vi "1.vi"() -> ()   [LabVIEW 2015]
panel:
  in  "OK Button":bool=TRUE
  in  "Requested Plots":T1(array[cluster])
  out "Waveform chart":waveform(dbl)[](graph)=[{"t0"=timestamp(3537897551.4112577 s since 1904-01-01), "dt"=1.0, "Y"=[1.0]}, {"t0"=timestamp(3537897551.411394 s since 1904-01-01), "dt"=1.0, "Y"=[52636.62109375]}, {"t0"=timestamp(3537897551.411678 s since 1904-01-01), "dt"=1.0, "Y"=[-339720.71875]}, {"t0"=timestamp(3537897551.411799 s since 1904-01-01), "dt"=1.0, "Y"=[202592.15625]}, {"t0"=timestamp(3537897551.4119 s since 1904-01-01), "dt"=1.0, "Y"=[-23028.4296875]}, {"t0"=timestamp(3537897551.411996 s since 1904-01-01), "dt"=1.0, "Y"=[88723.75]}, {"t0"=timestamp(3537897551.41212 s since 1904-01-01), "dt"=1.0, "Y"=[80100.75]}, {"t0"=timestamp(3537897551.310503 s since 1904-01-01), "dt"=1.0, "Y"=[-548105.4375]}]
  out "net address":u32
  out "port or service name":u16=5803
  in  "stop":bool
  out "error out":errorcluster
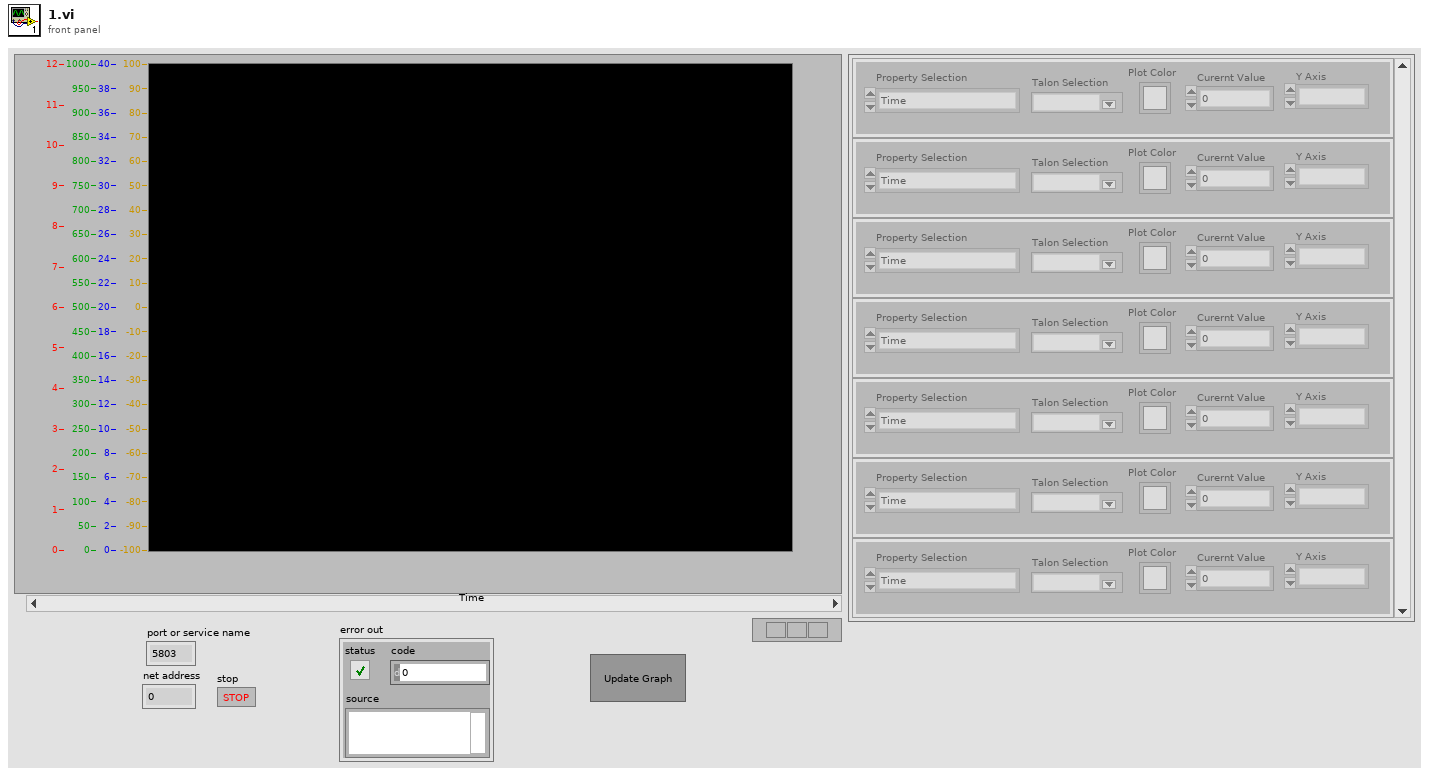
[diagram p1: front panel]
types:
  T1 = cluster{"Property Selection":enum16{"Time", "TalonID", "OutputVoltage", "OutputCurrent", "PIDError", "Encoder Position", "Encoder Velocity", "Commanded Value", "I Zone", "I Accumulation"}, "Talon Selection":u16, "Plot Color":u32, "Curernt Value":dbl, "New Current Value?":bool, "output waveform":waveform(dbl), "Y Axis":enum16{"Red Axis", "Green Axis", "Blue Axis", "Yellow Axis"}}[]
  T2 = enum16{"Red Axis", "Green Axis", "Blue Axis", "Yellow Axis"}[]
  T3 = enum16{"Time", "TalonID", "OutputVoltage", "OutputCurrent", "PIDError", "Encoder Position", "Encoder Velocity", "Commanded Value", "I Zone", "I Accumulation"}
  T4 = enum16{"Red Axis", "Green Axis", "Blue Axis", "Yellow Axis"}
  T5 = cluster{"Property Selection":enum16{"Time", "TalonID", "OutputVoltage", "OutputCurrent", "PIDError", "Encoder Position", "Encoder Velocity", "Commanded Value", "I Zone", "I Accumulation"}, "Talon Selection":u16, "Plot Color":u32, "Curernt Value":dbl, "New Current Value?":bool, "output waveform":waveform(dbl), "Y Axis":enum16{"Red Axis", "Green Axis", "Blue Axis", "Yellow Axis"}}
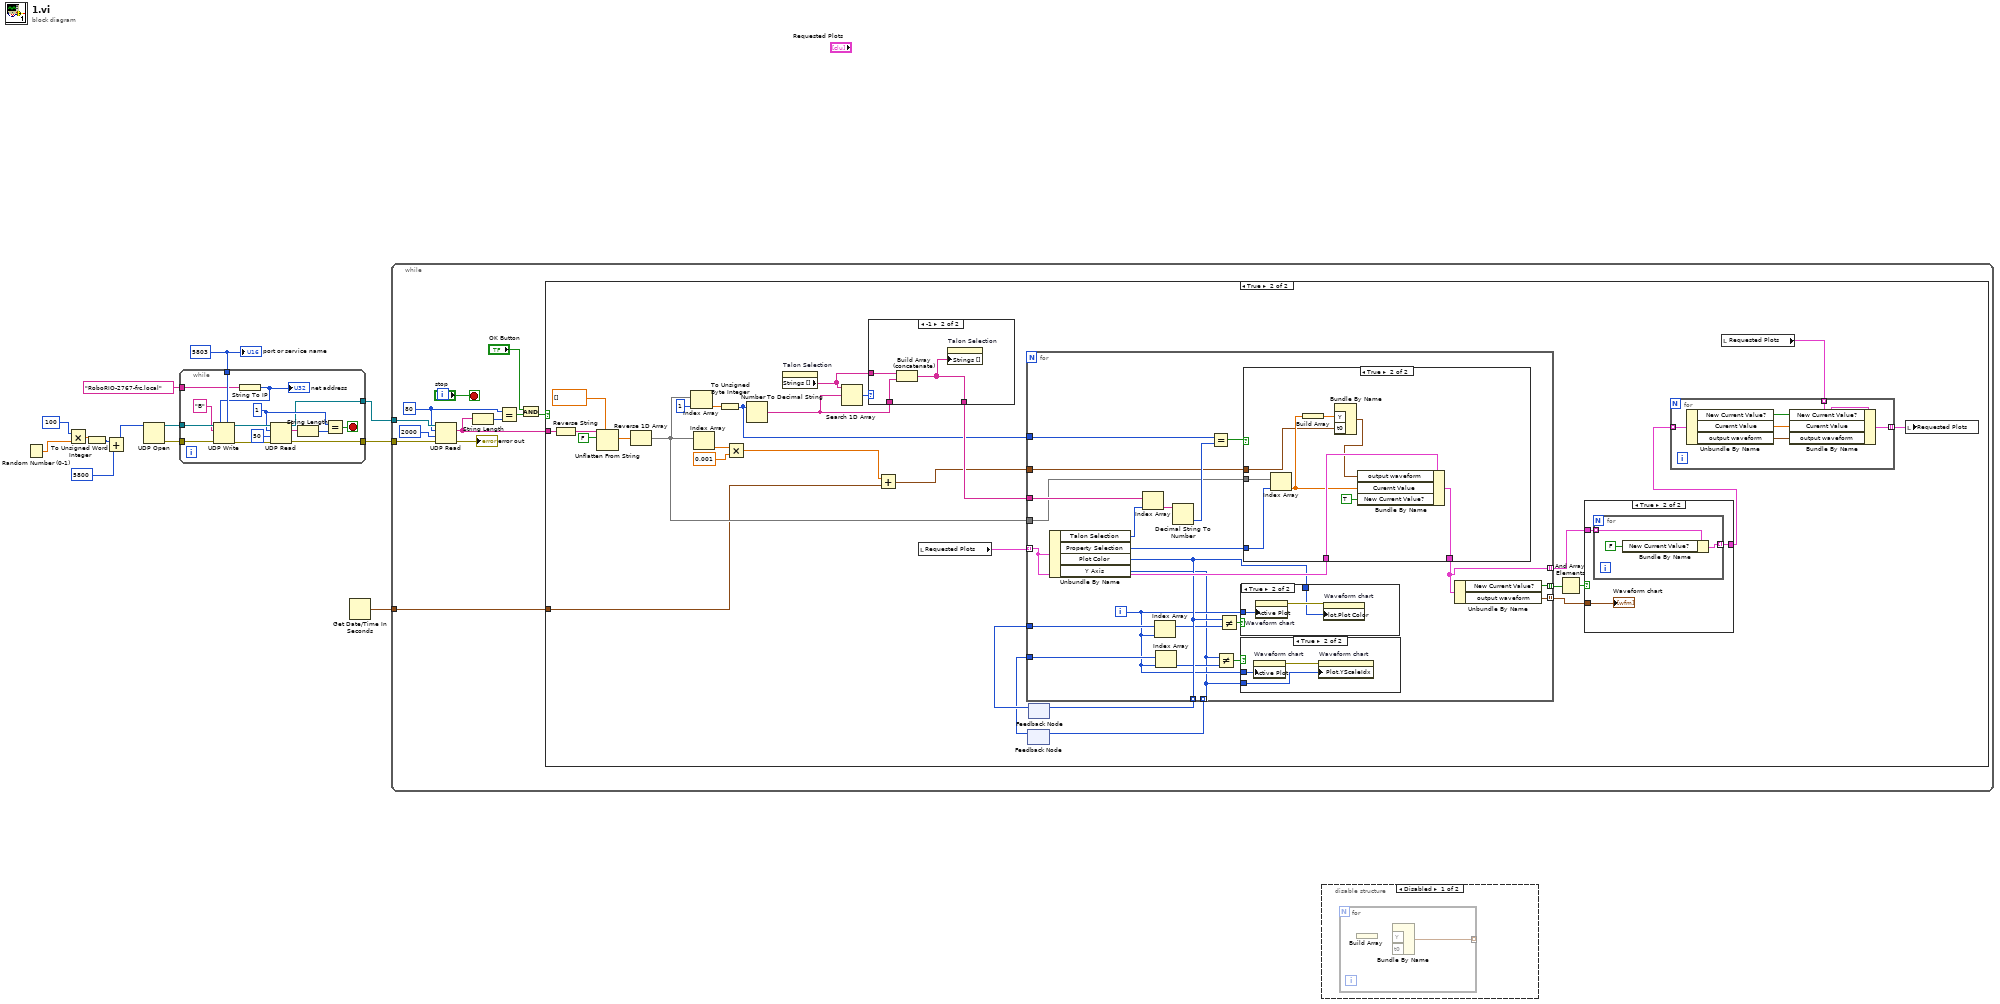
[diagram p0: block diagram]
diagram:
  w3 = u16 5803 ("port or service name")
  n1 = Random Number (0-1)() -> (number: 0 to 1=w7:dbl)
  n2 = Multiply(x=u16 100 ("port"), y=w7) -> (x*y=w6:dbl)
  n3 = To Unsigned Word Integer(number=w6) -> (unsigned 16bit integer=w5:u16)
  n4 = Add(x=w5, y=u16 5800 ("port")) -> (x+y=w9:u16)
  n5 = UDP Open(11:w9) -> (port=w13:refnum<k16>, 0:w12:errorcluster)  [unwired: 4 in, 1 out]
  n6 = while {
    tunnel: w13 -> [w28]
    tunnel: [w21] -> w4
    tunnel: w12 -> [w20]
    tunnel: [w19] -> w11
    tunnel: w3 -> [w17]
    tunnel: "RoboRIO-2767-frc.local" ("name") -> [w16]
    stop <- w22 stop-if-true
    w23 = 1 ("max size (548)")
    n7 = String To IP(1:w16) -> (0:w15:u32)
    "net address" <- w15
    n8 = UDP Write(address=w15, port or service name=w17, connection ID=w28, data in="B", 8:w20) -> (error out=w27:errorcluster, 3:w26:refnum<k16>)  [unwired: 1 in]
    n9 = UDP Read(connection ID=w26, max size (548)=w23, timeout ms (25000)=50, 8:w27) -> (data out=w25:string, error out=w19:errorcluster, 3:w21:refnum<k16>)  [unwired: 2 out]
    n10 = String Length(string=w25) -> (length=w24:i32)
    n11 = Equal?(x=w23, y=w24) -> (x = y?=w22:bool)
  }
  n12 = Get Date/Time In Seconds() -> (seconds since 1Jan1904=w1:timestamp)
  n13 = while {
    tunnel: w4 -> [w40]
    tunnel: w11 -> [w39]
    tunnel: w1 -> [w31]
    stop <- "stop" stop-if-true
    w33 = 80 ("max size (548)")
    n14 = UDP Read(connection ID=w40, max size (548)=w33, timeout ms (25000)=2000, 8:w39) -> (data out=w35:string, error out=→"error out":errorcluster)  [unwired: 3 out]
    n15 = String Length(string=w35) -> (length=w34:i32)
    n16 = Equal?(x=w33, y=w34) -> (x = y?=w32:bool)
    n17 = And(x="OK Button", y=w32) -> (x .and. y?=w30:bool)
    n18 = case shown="True" w30 {
      tunnel: w35 -> [_ w69]
      tunnel: w31 -> [_ w53]
      frame False {
      }
      frame True {
        n19 = Reverse String(1:w69) -> (0:w68:string)
        n20 = Unflatten From String(type=dbl[] [], binary string=w68, data includes array or string size? (T)=FALSE) -> (value=w66:dbl[])  [unwired: 2 in, 2 out]
        n21 = Reverse 1D Array(array=w66) -> (reversed array=w56:dbl[])
        n22 = Index Array(array=w56, index=1) -> (element=w62:dbl)
        n23 = Index Array(array=w56) -> (element=w65:dbl)  [unwired: 1 in]
        n24 = To Unsigned Byte Integer(number=w62) -> (unsigned 8bit integer=w57:u8)
        n25 = Multiply(x=w65, y=0.001) -> (x*y=w52:dbl)
        n26 = Number To Decimal String(number=w57) -> (decimal integer string=w59:string)  [unwired: 1 in]
        n27 = property on="Talon Selection" class="Ring (strict)"() -> ("Strings []"=w60:string[])  [unwired: 2 in, 2 out]
        n28 = Search 1D Array(1D array=w60, element=w59) -> (index of element=w61:i32)  [unwired: 1 in]
        n29 = case shown="-1" w61 {
          tunnel: w60 -> [w84 w86]
          tunnel: w59 -> [_ w87]
          tunnel: [w84 w85] -> w58
          frame 0, Default {
          }
          frame -1 {
            n30 = Build Array (concatenate)(w86, w87) -> (w85:string[])
            n31 = property on="Talon Selection" class="Ring (strict)"("Strings []"=w85) -> ()  [unwired: 2 in, 2 out]
          }
        }
        n32 = Add(x=w52, y=w53) -> (x+y=w54:timestamp)
        n33 = local read "Requested Plots"() -> (w49:T1)
        n34 = feedback #1() -> (w42:T2)  [unwired: 1 in]
        n35 = feedback #2() -> (w46:u32[])  [unwired: 1 in]
        n36 = for {
          tunnel: w49 -> [w101] mode=indexing
          tunnel: w58 -> [w108]
          tunnel: w57 -> [w106]
          tunnel: w56 -> [w102]
          tunnel: [w100] -> w55 mode=indexing
          tunnel: w54 -> [w99]
          tunnel: [w98] -> w50 mode=indexing
          tunnel: [w97] -> w48 mode=indexing
          tunnel: [w95] -> w47 mode=indexing
          tunnel: w46 -> [w93]
          tunnel: w42 -> [w92]
          tunnel: [w88] -> w41 mode=indexing
          i -> [w89]
          n37 = Unbundle By Name(w101) -> ("Talon Selection"=w109:u16, "Property Selection"=w103:T3, "Plot Color"=w95:u32, "Y Axis"=w88:T4)
          n38 = Index Array(array=w108, index=w109) -> (element=w107:string)
          n39 = Index Array(array=w93, index=w89) -> (element=w94:u32)
          n40 = Index Array(array=w92, index=w89) -> (element=w90:T4)
          n41 = Decimal String To Number(string=w107) -> (number=w105:i32)  [unwired: 2 in, 1 out]
          n42 = Equal?(x=w106, y=w105) -> (x = y?=w104:bool)
          n43 = Not Equal?(x=w88, y=w90) -> (x != y?=w91:bool)
          n44 = Not Equal?(x=w95, y=w94) -> (x != y?=w96:bool)
          n45 = case shown="True" w96 {
            tunnel: w89 -> [_ w114]
            tunnel: w95 -> [_ w113]
            frame False {
            }
            frame True {
              n46 = property on="Waveform chart" class="WFChart (strict)"("Active Plot"=w114) -> (error out=w115:errorcluster)  [unwired: 2 in, 1 out]
              n47 = property on="Waveform chart" class="WFChart (strict)"(error in=w115, "Plot.Plot Color"=w113) -> ()  [unwired: 1 in, 2 out]
            }
          }
          n48 = case shown="True" w91 {
            tunnel: w89 -> [_ w112]
            tunnel: w88 -> [_ w110]
            frame False {
            }
            frame True {
              n49 = property on="Waveform chart" class="WFChart (strict)"("Active Plot"=w112) -> (error out=w111:errorcluster)  [unwired: 2 in, 1 out]
              n50 = property on="Waveform chart" class="WFChart (strict)"(error in=w111, "Plot.YScaleIdx"=w110) -> ()  [unwired: 1 in, 2 out]
            }
          }
          n51 = case shown="True" w104 {
            tunnel: w103 -> [_ w124]
            tunnel: w102 -> [_ w125]
            tunnel: w101 -> [w116 w123]
            tunnel: [w116 w122] -> w97
            tunnel: w99 -> [_ w117]
            frame False {
            }
            frame True {
              n52 = Index Array(array=w125, index=w124) -> (element=w119:dbl)
              n53 = Build Array(w119) -> (w118:dbl[])
              n54 = Bundle By Name("Y"=w118, "t0"=w117) -> (w120:waveform(dbl))  [unwired: 1 in]
              n55 = Bundle By Name(cluster=w123, "output waveform"=w120, "Curernt Value"=w119, "New Current Value?"=TRUE) -> (w122:T5)
            }
          }
          n56 = Unbundle By Name(w97) -> ("New Current Value?"=w100:bool, "output waveform"=w98:waveform(dbl))
        }
        n57 = feedback-in #1(w41) -> ()
        n58 = feedback-in #2(w47) -> ()
        n59 = And Array Elements(Boolean array=w55) -> (logical AND=w51:bool)
        n60 = case shown="True" w51 {
          tunnel: w50 -> [_ w80]
          tunnel: w48 -> [w77 w79]
          tunnel: [w77 w78] -> w43
          frame False {
          }
          frame True {
            n61 = for {
              tunnel: w79 -> [w83] mode=indexing
              tunnel: [w81] -> w78 mode=indexing
              n62 = Bundle By Name(cluster=w83, "New Current Value?"=FALSE) -> (w81:T5)
            }
            "Waveform chart" <- w80
          }
        }
        n63 = local read "Requested Plots"() -> (w44:T1)
        n64 = for {
          tunnel: [w75] -> w45 mode=indexing
          tunnel: w44 -> [w76] mode=indexing
          tunnel: w43 -> [w71] mode=indexing
          n65 = Unbundle By Name(w71) -> ("New Current Value?"=w74:bool, "Curernt Value"=w73:dbl, "output waveform"=w72:waveform(dbl))
          n66 = Bundle By Name(cluster=w76, "New Current Value?"=w74, "Curernt Value"=w73, "output waveform"=w72) -> (w75:T5)
        }
        n67 = local write "Requested Plots"(w45) -> ()
      }
    }
  }
  n68 = disable-structure shown="Disabled" {
    frame Disabled {
      n69 = for {
        tunnel: [w126] -> _ mode=indexing
        n70 = Build Array() -> ()  [unwired: 1 in, 1 out]
        n71 = Bundle By Name() -> (w126:waveform(dbl))  [unwired: 3 in]
      }
    }
    frame Enabled {
    }
  }
  "port or service name" <- w3
